vi "About.vi"() -> ()   [LabVIEW 2014]
panel:
  in  "OK Button":bool
  # "此遊戲是模擬噬謊者這本漫畫中出現的遊戲Air Poker來製作，有看過漫畫的人應該可以看出\n跟漫畫還有一點不同，所以強烈推薦沒看過這本漫畫的人去看，神作!反正剛好最近疫情原因，可以殺殺時間?"
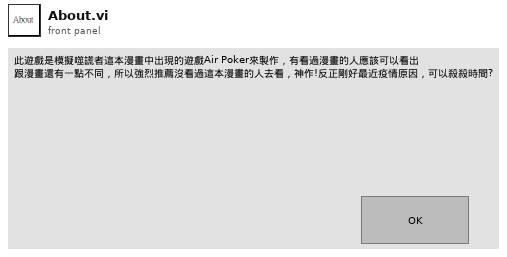
[diagram p1: front panel]
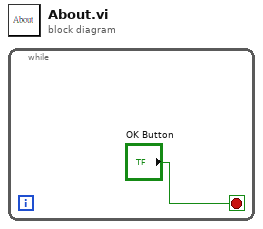
[diagram p0: block diagram]
diagram:
  n1 = while {
    stop <- "OK Button" stop-if-true
  }
